vi "RT Main.vi"() -> ()   [LabVIEW 2019]
doc: "The myRIO Custom FPGA Project template acquires button data from the onboard button and displays the button value on a Boolean indicator. The SYS.RDY indicator shows the FPGA status."
uses:
  <vilib>/FPGAPlugInAG/myRIO-1900/niLvFpga_Open_myRIO-1900.vi
  <vilib>/rvi/interface/common/dynamic/niFpgaDynamicAddResources.vi
  <vilib>/Utility/error.llb/Error Cluster From Error Code.vi
  <vilib>/rvi/errors/niLvFpgaAdjustHostInterfaceError.vi
  <vilib>/rvi/interface/nirviOpenFPGA/nirviOpenFPGA.xnode
  FPGA Bitfiles/hybridpulser_FPGATarget_fpgamainfsm_024CIbEM8OY.lvbitx
  <vilib>/rvi/interface/nirviMethod/nirviMethod.xnode
  <vilib>/FPGAPlugInAG/Dynamic/niLvFpga_WriteFifo_Dynamic.vi
  <vilib>/rvi/errors/niLvFpgaMergeErrorWithErrorCode.vi
panel:
  in  "data":u32[](array[numeric])
  in  "cmd":u8[](array[numeric])
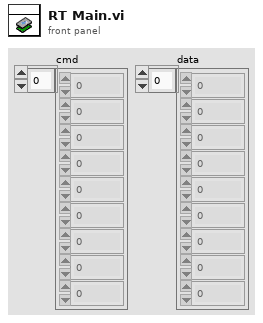
[diagram p1: front panel]
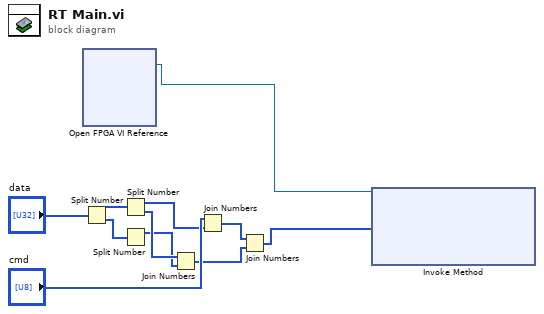
[diagram p0: block diagram]
diagram:
  n1 = Split Number(x="data") -> (hi(x)=w8:u16[], lo(x)=w9:u16[])
  n2 = xnode "Open FPGA VI Reference"() -> ("FPGA VI Reference Out"=w11:refnum<k20>)  [unwired: 2 in, 1 out]
  n3 = Split Number(x=w8) -> (hi(x)=w6:u8[], lo(x)=w5:u8[])
  n4 = Split Number(x=w9) -> (hi(x)=w4:u8[])  [unwired: 1 out]
  n5 = Join Numbers(hi=w5, lo=w4) -> ((hi.lo)=w2:u16[])
  n6 = Join Numbers(hi="cmd", lo=w6) -> ((hi.lo)=w3:u16[])
  n7 = Join Numbers(hi=w3, lo=w2) -> ((hi.lo)=w1:u32[])
  n8 = xnode "Invoke Method"("FPGA VI Reference In"=w11, "Data"=w1) -> ()  [unwired: 2 in, 3 out]
